vi "Test In-Range Greyscale Image.vi"(8 "error in (no error)":errorcluster, 11 "Test Case In":refnum<class "01_Image.lvclass">) -> (0 "error out":errorcluster, 3 "Test Case Out":refnum<class "01_Image.lvclass">)   [LabVIEW 2020, in "test.lvlib" / "01_Image.lvclass"]
uses:
  01_Image.lvclass
  C:/Program Files (x86)/National Instruments/LabVIEW 2026/vi.lib/Astemes/LUnit/Test Case.lvclass
  common/Image Size (Integer).ctl
  image/In-Range Image Grey Range.ctl
  <vilib>/Astemes/LUnit/Test Case.lvclass/Test Case.ctl
  image/New Image (Greyscale Preallocated).vi
  4993e8ee-a06a-463a-9684-69129f64d5ce.vi
  image/Copy Array to Image.vi
  image/Copy Array to Image (Greyscale).vi
  image/New Image (Greyscale Preallocated).vi/6598b9e0-8a08-46f5-91fd-ca1b87217137.vi
  image/In-Range (Greyscale).vi/5701baee-35e2-4306-9a77-a9fdbb5b3a7f.vi
  <vilib>/Astemes/LUnit/Core/LUnit Test Case/Private/Append Pass Result.vi
  <vilib>/Astemes/LUnit/Core/LUnit Test Case/Private/Append Fail Result.vi
  4993e8ee-a06a-463a-9684-69129f64d5ce.vi/9c5d11cd-9439-4240-a1ee-d9baace9c924.vi
  <vilib>/Astemes/LUnit/Core/LUnit Test Case/Private/Run In UI.vi
  <vilib>/Utility/error.llb/Clear Errors.vi
  <vilib>/Utility/error.llb/Error Cluster From Error Code.vi
  <vilib>/picture/pixmap.llb/Flatten Pixmap.vi
  image/image.lvlib
  common/common.lvlib
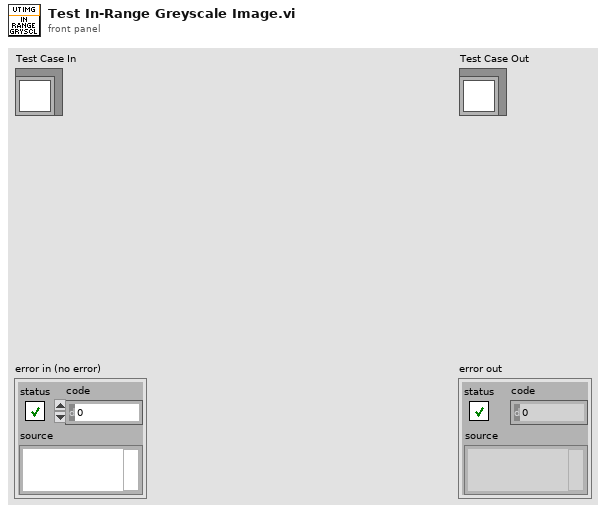
[diagram p1: front panel]
types:
  T1 = typedef "image.lvlib/In-Range Image Grey Range.ctl" = cluster{"Lower":u8, "Upper":u8}
  T2 = typedef "common.lvlib/Image Size (Integer).ctl" = cluster{"Width":u16, "Height":u16}
  T3 = typedef "image.lvlib/Greyscale Image.ctl" = refnum<data-value>
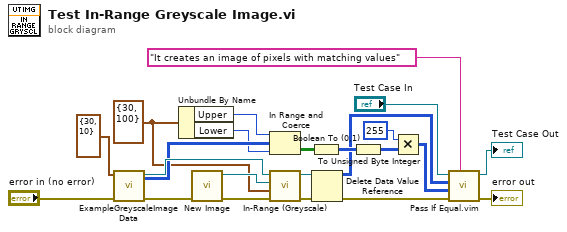
[diagram p0: block diagram]
diagram:
  w9 = T1 {"Lower"=30, "Upper"=100} ("In-Range Image Colour Range")
  n1 = call "ExampleGreyscaleImageData.vi"("error in (no error)"="error in (no error)", "Image Size"=T2 {"Width"=30, "Height"=10} ("Preallocated Image Size (Default - 0,0)")) -> ("error out"=w18:errorcluster, "Greyscale Destination Image"=w11:T3, "Greyscale Data"=w10:u8[][])  [unwired: 6 in, 1 out]
  n2 = Unbundle By Name(w9) -> ("Upper"=w7:u8, "Lower"=w8:u8)
  n3 = call-poly "New Image.vi"("error in (no error)"=w18) -> ("error out"=w17:errorcluster, "Greyscale Image"=w13:T3)  [unwired: 9 in]
  n4 = In Range and Coerce(upper limit=w7, x=w10, lower limit=w8) -> (In Range?=w6:bool[][])  [unwired: 1 out]
  n5 = call "In-Range (Greyscale).vi"("error in (no error)"=w17, "In-Range Image Colour Range"=w9, "In-Range-Result in"=w13, "Greyscale Image-Source in"=w11) -> ("error out"=w14:errorcluster, "In-Range-Result"=w12:T3)  [unwired: 6 in]
  n6 = Boolean To (0,1)(Boolean=w6) -> (0, 1=w5:i16[][])
  n7 = Delete Data Value Reference(data value reference=w12, error in=w14) -> (data value=w3:u8[][], error out=w16:errorcluster)
  n8 = To Unsigned Byte Integer(number=w5) -> (unsigned 8bit integer=w1:u8[][])
  n9 = Multiply(x=u8 255, y=w1) -> (x*y=w2:u8[][])
  n10 = call "Pass If Equal.vim"("Description"="It creates an image of pixels with matching values", "error in (no error)"=w16, "Actual"=w2, "Expected"=w3, "LUnit Test Case In"="Test Case In") -> ("error out"=→"error out":errorcluster, "LUnit Test Case Out"=→"Test Case Out":refnum<class "01_Image.lvclass">)  [unwired: 5 in]
